vi "testcluster.vi"() -> ()   [LabVIEW 2023]
uses:
  High Level Capabilities/Chiller/Chiller.lvclass
  Utilities/Utilities.lvlib
panel:
  out "JSON string":string
  in  "ChillerConsumerChannels":T1
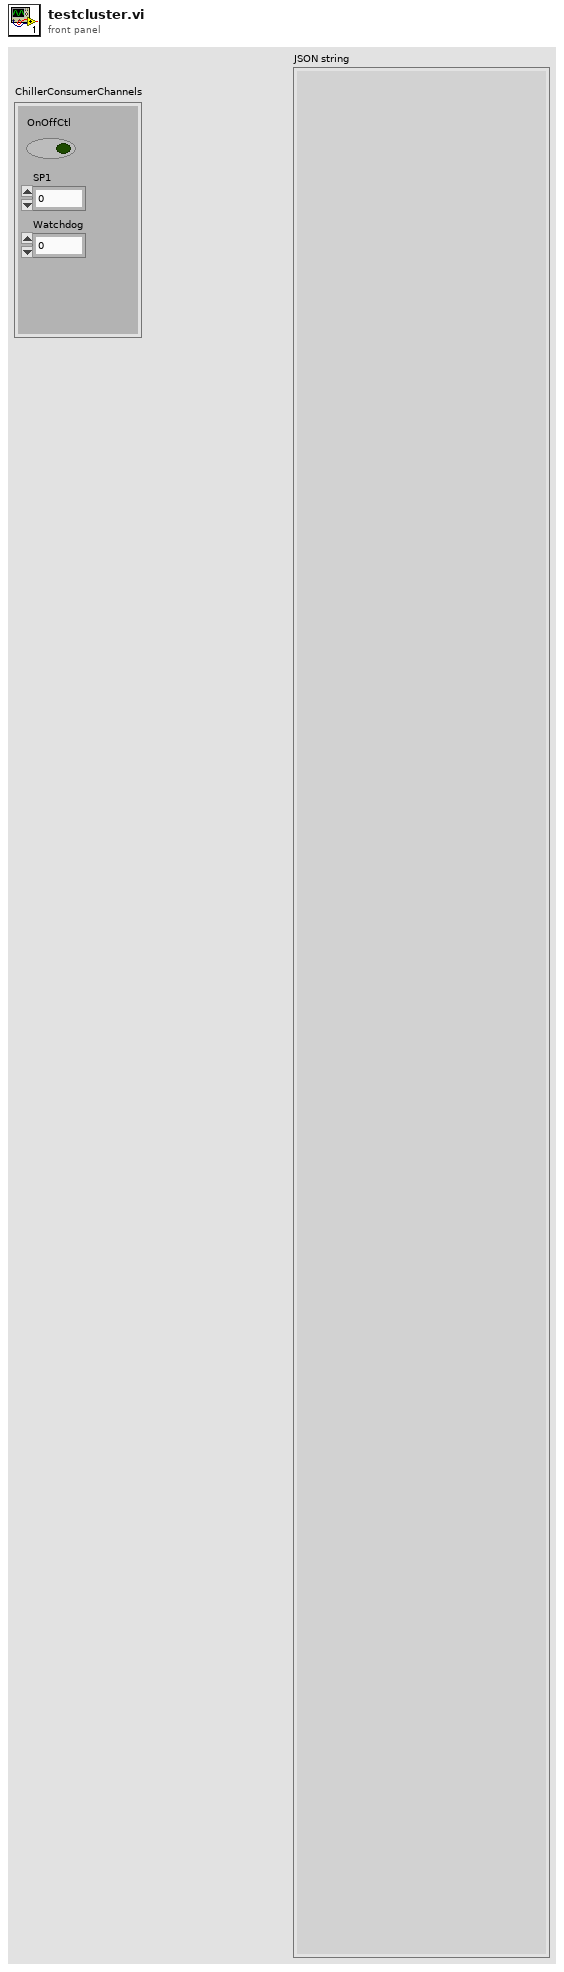
[diagram p1: front panel]
types:
  T1 = cluster{"OnOffCtl":bool, "SP1":i32, "Watchdog":dbl}
  T2 = typedef "Utilities.lvlib/Channel.ctl" = cluster{"Consumer?":bool, "Title":string, "Name":string, "Description":string, "Size":i32, "OffSets":i32[], "SubTitle":string[], "DataType":string[]}
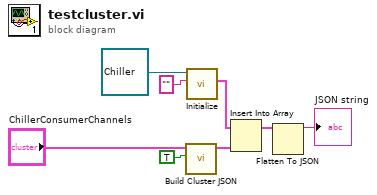
[diagram p0: block diagram]
diagram:
  n1 = call "Build Cluster JSON.vi"("Consumer?"=TRUE, "Cluster"="ChillerConsumerChannels") -> ("Channel"=w3:T2)  [unwired: 9 in]
  n2 = call-dynamic "Initialize.vi"("Instance Name"="", "Chiller in"=refnum<class "Chiller.lvclass"> refnum) -> ("Channel"=w4:T2[])  [unwired: 7 in, 2 out]
  n3 = Insert Into Array(array=w4, new element=w3) -> (w5:T2[])  [unwired: 1 in]
  n4 = Flatten To JSON(anything=w5) -> (JSON string=→"JSON string":string)  [unwired: 2 in, 1 out]
